vi "Cost.vi"(8 "error in (no error)":errorcluster, 11 "Beverage in":refnum<class "Beverage.lvclass">) -> (0 "error out":errorcluster, 2 "Cost":dbl, 3 "Beverage out":refnum<class "Beverage.lvclass">)   [LabVIEW 2011, in "Beverage.lvclass"]
uses:
  Beverage.lvclass
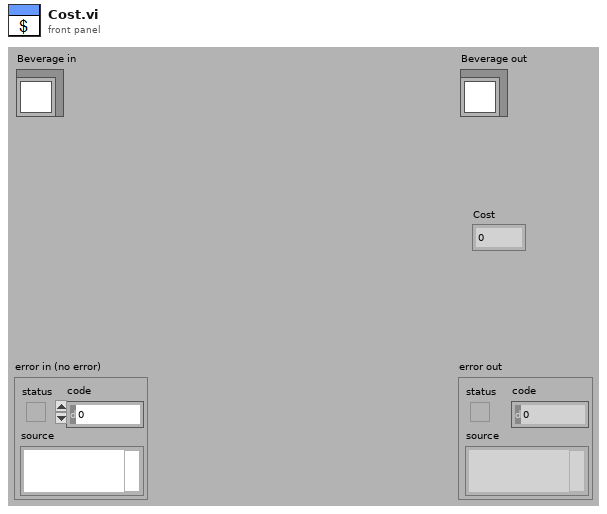
[diagram p1: front panel]
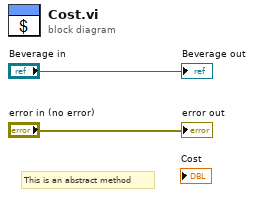
[diagram p0: block diagram]
diagram:
  # "This is an abstract method"
  "error out" <- "error in (no error)"
  "Beverage out" <- "Beverage in"
